vi "Get Core Count.vi"(8 "error in (no error)":errorcluster, 11 "CPU Info in":refnum<class "CPU Hardware Info.lvclass">) -> (0 "error out":errorcluster, 2 "Core Count":i32, 3 "CPU Info out":refnum<class "CPU Hardware Info.lvclass">)   [LabVIEW 2017, in "Data Sharing Framework Engine.lvlib" / "CPU Hardware Info.lvclass"]
uses:
  CPU Hardware Info.lvclass
  CPU Hardware Info.lvclass/CPU Hardware Info.ctl
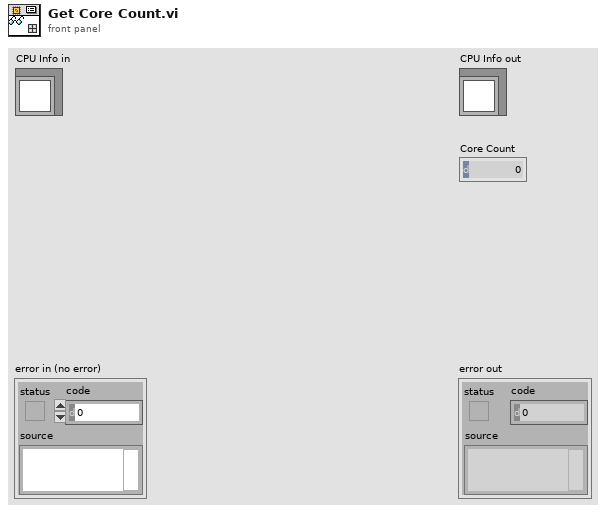
[diagram p1: front panel]
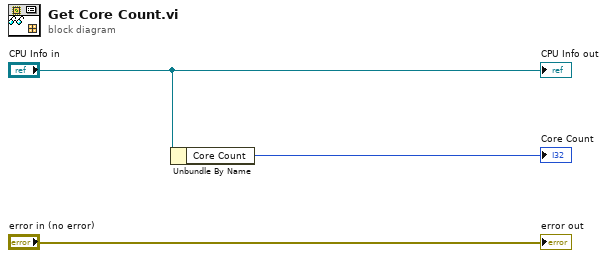
[diagram p0: block diagram]
diagram:
  n1 = Unbundle By Name("CPU Info in") -> ("Core Count"=→"Core Count":i32)
  "error out" <- "error in (no error)"
  "CPU Info out" <- "CPU Info in"
